vi "Bar.vi"() -> (0 "Numeric":i32, 1 "Time Out Value":u8, 2 "Barcode Scane":bool, 3 "Out":bool)   [LabVIEW 2015]
uses:
  Control Button/Exit.ctl
  Control PB/Next_.ctl
panel:
  in  "Barcode Scaner Selection":enum16{"MIC Barcode "}(ring)
  in  "Time Out (ms)":u32
  in  "Barcode":bool
  in  "Next":T1
  in  "Exit":T2
  # "Add Feature List"
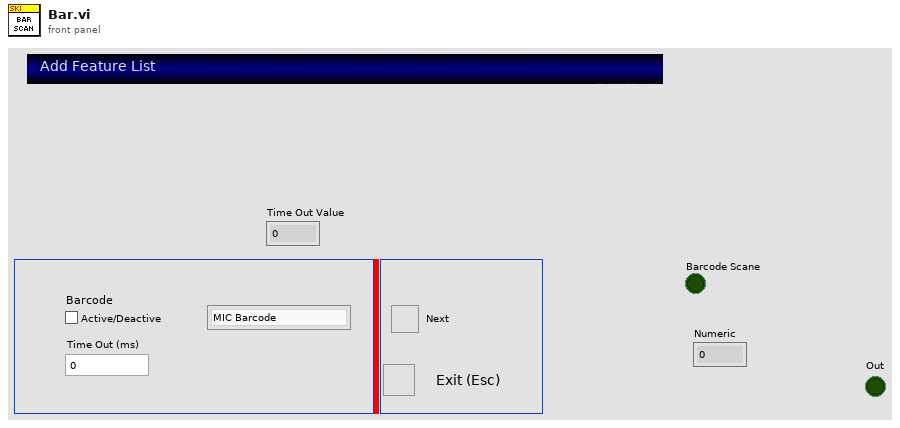
[diagram p1: front panel]
types:
  T1 = typedef "Next_.ctl" = bool
  T2 = typedef "Exit.ctl" = bool
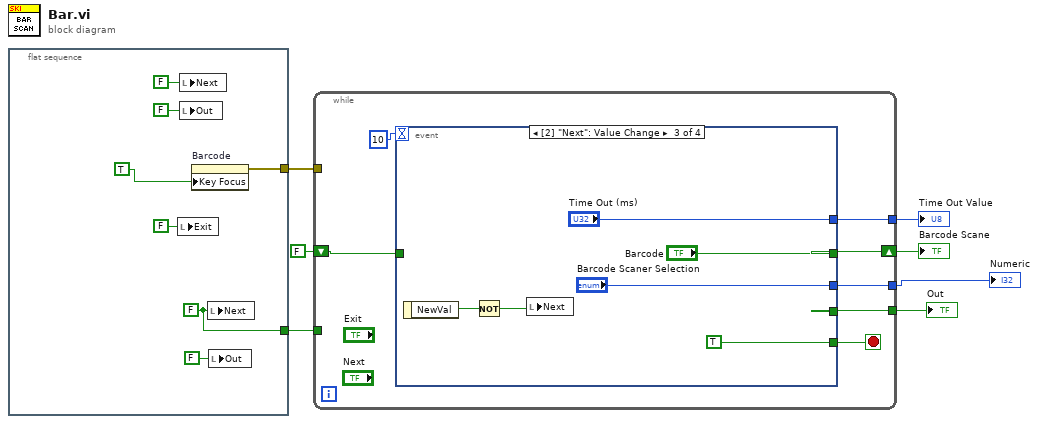
[diagram p0: block diagram]
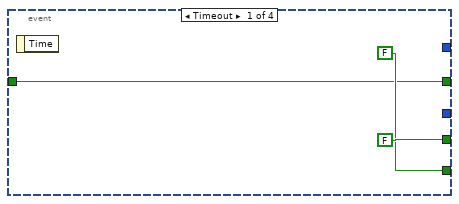
[diagram p2: hidden frame]
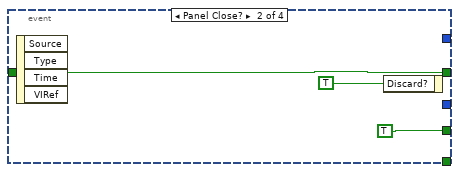
[diagram p3: hidden frame]
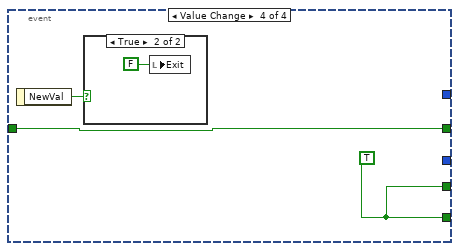
[diagram p4: hidden frame]
diagram:
  n1 = flat-sequence {
    tunnel: [w11] -> w6
    tunnel: [w8] -> w5
    frame #0 {
      w11 = T1 FALSE ("Next")
      n2 = local write "Exit"(FALSE ("Exit")) -> ()
      n3 = local write "Next"(T1 FALSE ("Next")) -> ()
      n4 = local write "Out"(FALSE ("Out")) -> ()
      n5 = property on="Barcode" class="Bool (strict)"("Key Focus"=TRUE) -> (error out=w8:errorcluster)  [unwired: 2 in, 1 out]
      n6 = local write "Next"(w11) -> ()
      n7 = local write "Out"(FALSE ("Out")) -> ()
    }
  }
  n8 = while {
    tunnel: [w19] -> w7
    tunnel: w6 -> [_]
    shift-right: [w20] -> w4
    shift-left: FALSE ("Barcode") -> [w17]
    tunnel: w5 -> [_]
    tunnel: [w16] -> w3
    tunnel: [w15] -> w1
    stop <- w21 stop-if-true
    n9 = event shown="[2] \"Next\": Value Change" {
      selector: _ -> [_ _ _ _]
      dyn-events: _ -> [_ _ _ _]
      timeout: 10 -> [_ _ _ _]
      tunnel: [FALSE _ T1 TRUE ("NewVal") w34] -> w21
      tunnel: [w22 w25 "Barcode" w35] -> w20
      tunnel: [T1 FALSE ("NewVal") T1 TRUE ("NewVal") _ w34] -> w19
      tunnel: w17 -> [w22 w25 _ w35]
      tunnel: [_ _ "Time Out (ms)" _] -> w16
      tunnel: [_ _ "Barcode Scaner Selection" _] -> w15
      event Timeout {
        n10 = event-data() -> ()  [unwired: 1 in, 1 out]
      }
      event Panel Close? {
        n11 = event-data() -> ()  [unwired: 1 in, 4 out]
        n12 = event-data("Discard?"=TRUE) -> ()  [unwired: 1 in, 1 out]
      }
      event Value Change {
        n13 = event-data() -> ("NewVal"=w30:T1)  [unwired: 1 in]
        n14 = Not(x=w30) -> (.not. x?=w29:T1)
        n15 = local write "Next"(w29) -> ()
      }
      event Value Change {
        w34 = TRUE
        n16 = event-data() -> ("NewVal"=w36:T2)  [unwired: 1 in]
        n17 = case shown="True" w36 {
          frame False {
          }
          frame True {
            n18 = local write "Exit"(T1 FALSE ("Next")) -> ()
          }
        }
      }
    }
  }
  "Out" <- w7
  "Barcode Scane" <- w4
  "Time Out Value" <- w3
  "Numeric" <- w1
